vi "Write ModuleHeight.vi"(8 "error in (no error)":errorcluster, 10 "ModuleHeight":u8=10, 11 "Linear Barcode in":refnum<class "Linear Barcode.lvclass">) -> (0 "error out":errorcluster, 3 "Linear Barcode out":refnum<class "Linear Barcode.lvclass">)   [LabVIEW 2013, in "BarCodes.lvlib" / "Linear Barcode.lvclass"]
uses:
  Linear Barcode.lvclass
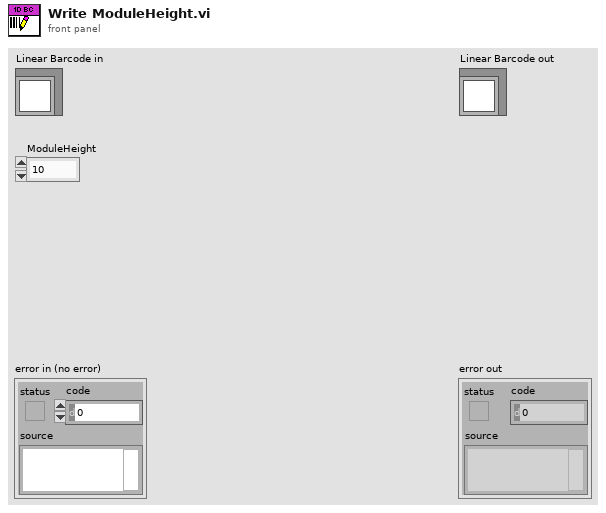
[diagram p1: front panel]
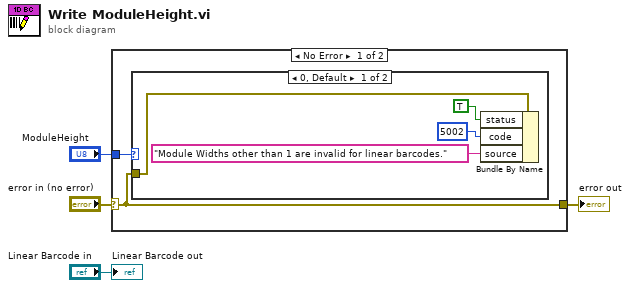
[diagram p0: block diagram]
diagram:
  n1 = case shown="No Error" "error in (no error)" {
    selector: "error in (no error)" -> [w6 w11]
    tunnel: [w6 w11] -> w4
    tunnel: "ModuleHeight" -> [w5 _]
    frame No Error {
      n2 = case shown="0, Default" w5 {
        tunnel: w6 -> [w10 _]
        frame 0, Default {
          n3 = Bundle By Name(cluster=w10, "status"=TRUE, "code"=5002, "source"="Module Widths other than 1 are invalid for linear barcodes.") -> ()  [unwired: 1 out]
        }
        frame 1 {
        }
      }
    }
    frame Error {
    }
  }
  "error out" <- w4
  "Linear Barcode out" <- "Linear Barcode in"
